vi "WPI_SPIClose.vi"(8 "error in (no error)":errorcluster, 11 "SPIDevRef":T1) -> (0 "error out":errorcluster)   [LabVIEW 2017]
doc: "Closes a reference to the SPI Engine. Use this VI to close each SPI reference that you open with the Open VI.\n\nThis software is licensed. Open the labview\\readme\\WPI Robotics Library Open Source License.txt file for more information."
uses:
  <vilib>/Rock Robotics/WPI/SPI/WPI_SPIDevRef.ctl
  <vilib>/Rock Robotics/SystemInterfaces/spilib/spi_bus.ctl
  <vilib>/Rock Robotics/WPI/SPI/WPI_SPIBusCacheOp.ctl
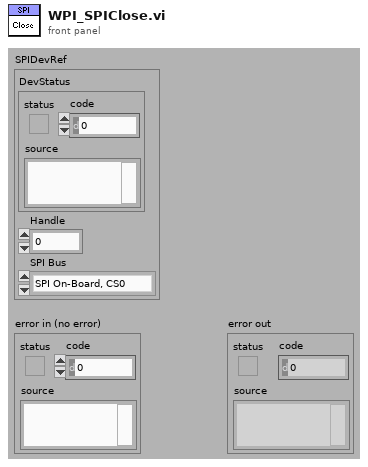
[diagram p1: front panel]
types:
  T1 = typedef "WPI_SPIDevRef.ctl" = cluster{"DevStatus":errorcluster, "Handle":i32, "SPI Bus":T2}
  T2 = typedef "spi_bus.ctl" = enum16{"SPI On-Board, CS0", "SPI On-Board, CS1", "SPI On-Board, CS2", "SPI On-Board, CS3", "SPI MXP", "Invalid"}
  T3 = typedef "WPI_SPIBusCacheOp.ctl" = enum16{"Acquire", "Release", "Status"}
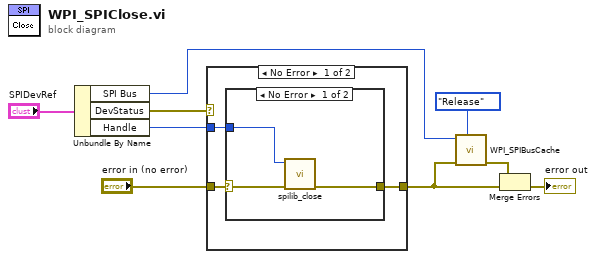
[diagram p0: block diagram]
diagram:
  n1 = Unbundle By Name("SPIDevRef") -> ("SPI Bus"=w1:T2, "DevStatus"=w7:errorcluster, "Handle"=w6:i32)
  n2 = case shown="No Error" w7 {
    selector: w7 -> [_ w17]
    tunnel: "error in (no error)" -> [w12 _]
    tunnel: [w11 w17] -> w5
    tunnel: w6 -> [w10 _]
    frame No Error {
      n3 = case shown="No Error" w12 {
        selector: w12 -> [w15 w16]
        tunnel: [w14 w16] -> w11
        tunnel: w10 -> [w13 _]
        frame No Error {
          n4 = call <vilib>:"spilib_close.vi"("error in (no error)"=w15, "handle"=w13) -> ("error out"=w14:errorcluster)  [unwired: 9 in]
        }
        frame Error {
        }
      }
    }
    frame Error {
    }
  }
  n5 = call <vilib>:"WPI_SPIBusCache.vi"("Operation"=WPI_SPIBusCacheOp."Release", "error in (no error)"=w5, "SPI Bus"=w1) -> ("error out"=w3:errorcluster)  [unwired: 6 in, 2 out]
  n6 = Merge Errors(w3, w5) -> (→"error out":errorcluster)
